vi "ROI entry-Offset all ROI.vi"(9 "Y offset":i8, 11 "X offset":i8) -> (0 "error out":errorcluster)   [LabVIEW 2013]
uses:
  Typedefs/Offsets cluster.ctl
  Typedefs/ROI management FG states.ctl
  Globals/gl_ROI Entry UI globals.vi
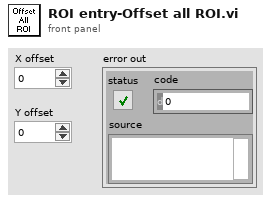
[diagram p1: front panel]
types:
  T1 = typedef "Offsets cluster.ctl" = cluster{"X offset":i8, "Y offset":i8}
  T2 = typedef "ROI entry screen ctrl refs cluster.ctl" = cluster{"Done button":refnum<vi>, "Imaging button":refnum<vi>, "Acquisition button":refnum<vi>, "POI dwell time (us)":refnum<vi>, "Scan dwell time per pixel (us)":refnum<vi>, "# of planes":refnum<vi>, "Zoom":refnum<vi>, "Equal size":refnum<vi>, "Channel":refnum<vi>, "Image Display":refnum<vi>, "Z-Plane Selector":refnum<vi>, "Number of lines left":refnum<vi>, "Z-stack folder path":refnum<vi>, "POI Density":refnum<vi>, "Arb Plane Entry":refnum<vi>, "Whole plane":refnum<vi>, "Clear Last":refnum<vi>, "Clear All":refnum<vi>, "Trial Length (sec)":refnum<vi>, "Palette Type":refnum<vi>, "Intensity slider":refnum<vi>, "# POI":refnum<vi>, "Max Z Proj":refnum<vi>, "Zplane ind":refnum<vi>, "Wavelength (nm)":refnum<vi>, "Number of Trials":refnum<vi>, "Funct stim.trig.enable":refnum<vi>, "Funct stim.trig.delay (s)":refnum<vi>, "Line Mode":refnum<vi>, "Step size (µm)":refnum<vi>, "ROI move mode":refnum<vi>, "Cool-down time (s)":refnum<vi>, "Enable cool-down time":refnum<vi>, "Motor Z ind. (um)":refnum<vi>, "AOL Z ind. (um)":refnum<vi>}
  T3 = typedef "ROI move mode.ctl" = enum16{"ROI on ALL planes", "ROI on current plane"}
  T4 = typedef "ROI management FG states.ctl" = enum16{"Read", "Write", "Clear Last", "Clear All", "Update ROIs time", "Reload last ROI set", "Offset all ROI", "Offset visible ROI"}
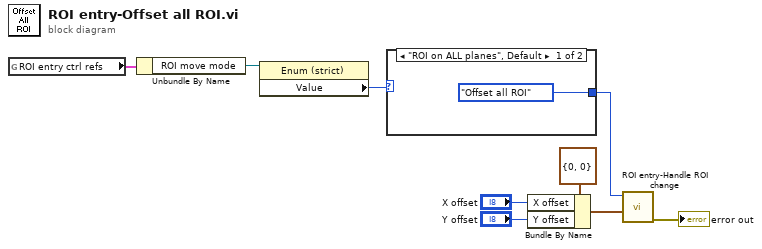
[diagram p0: block diagram]
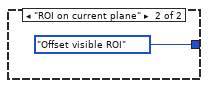
[diagram p2: hidden frame]
diagram:
  n1 = global read "gl_ROI Entry UI globals.vi" "ROI entry ctrl refs"() -> (w4:T2)
  n2 = Unbundle By Name(w4) -> ("ROI move mode"=w3:refnum<vi>)
  n3 = property class="Enum (strict)"(reference=w3) -> ("Value"=w2:T3)  [unwired: 1 in, 2 out]
  n4 = case shown="\"ROI on ALL planes\", Default" w2 {
    tunnel: [ROI_management_FG_states."Offset all ROI" ("Function") ROI_management_FG_states."Offset visible ROI" ("Function")] -> w1
    frame "ROI on ALL planes", Default {
    }
    frame "ROI on current plane" {
    }
  }
  n5 = Bundle By Name(cluster=T1 {"X offset"=0, "Y offset"=0} ("Offsets cluster"), "X offset"="X offset", "Y offset"="Y offset") -> (w8:T1)
  n6 = call "ROI entry-Handle ROI change.vi"("Offsets cluster"=w8, "ROI management"=w1) -> ("error out"=→"error out":errorcluster)  [unwired: 7 in, 2 out]
